vi "界面.vi"() -> ()   [LabVIEW 2024]
panel:
  in  "出错":string
  out "回答框":string
  in  "词数":dbl(slide)=50.38167938931298 scale=0.0..200.0
  in  "空白按钮":bool
  in  "发送":bool
  in  "输入框":string
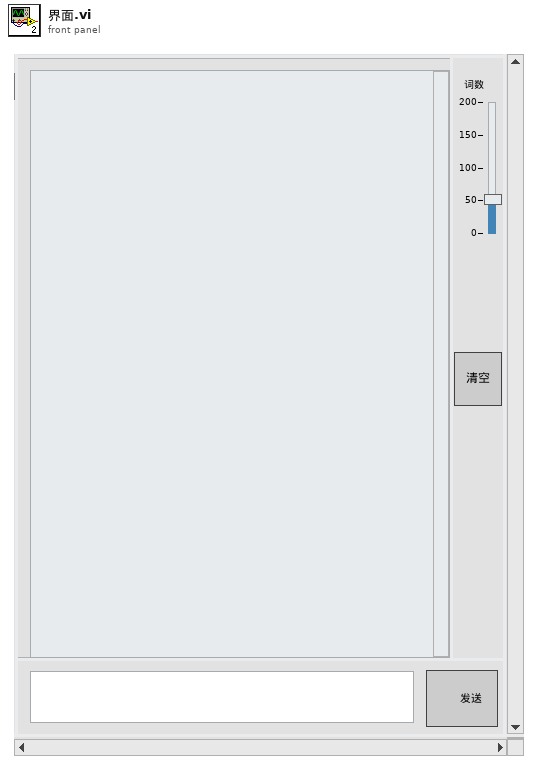
[diagram p1: front panel]
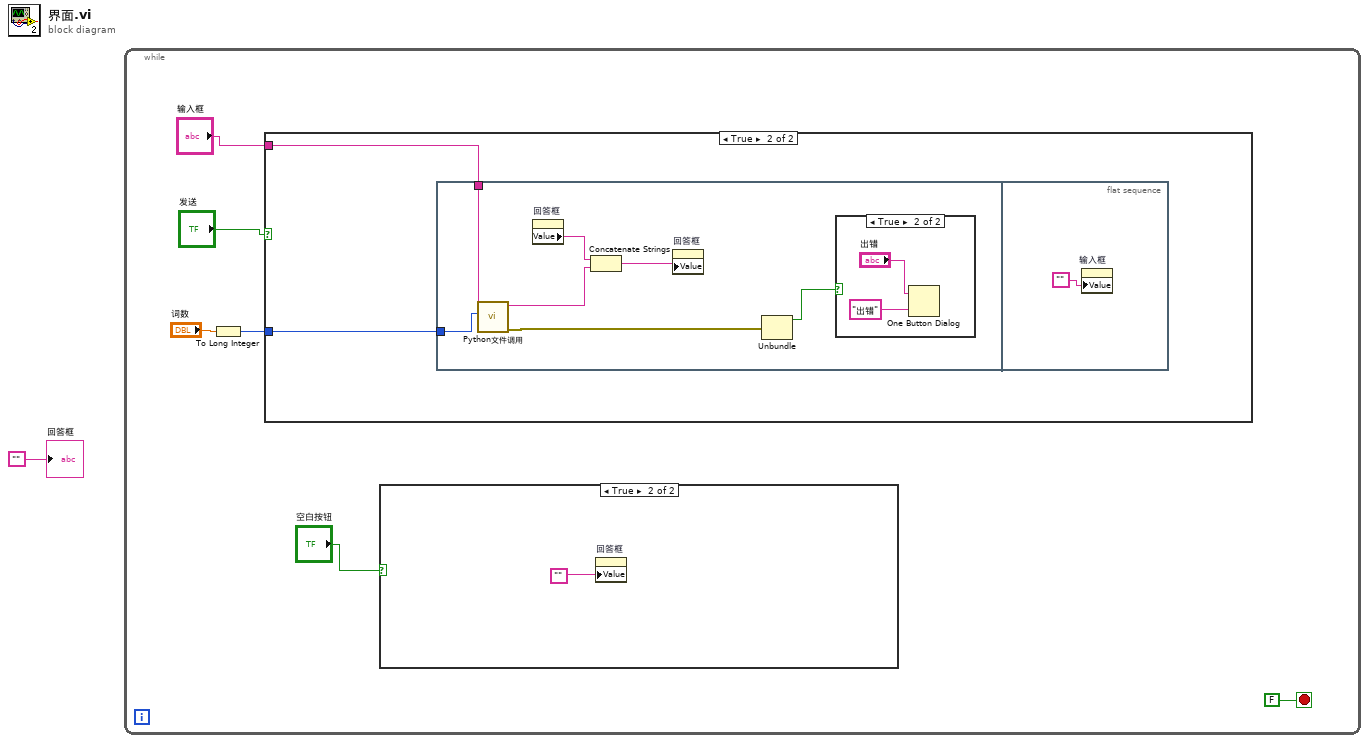
[diagram p0: block diagram]
diagram:
  n1 = while {
    stop <- FALSE stop-if-true
    n2 = To Long Integer(number="词数") -> (32bit integer=w2:i32)
    n3 = case shown="True" "发送" {
      tunnel: "输入框" -> [_ w10]
      tunnel: w2 -> [_ w9]
      frame False {
      }
      frame True {
        n4 = flat-sequence {
          tunnel: w10 -> [w17]
          tunnel: w9 -> [w11]
          frame #0 {
            n5 = call "Python文件调用.vi"("max_new_tokens"=w11, "text"=w17) -> ("错误输出"=w16:errorcluster, "out"=w13:string)  [unwired: 8 in]
            n6 = property on="回答框" class="Str"() -> ("Value"=w14:string)  [unwired: 2 in, 2 out]
            n7 = Concatenate Strings(w14, w13) -> (w12:string)
            n8 = property on="回答框" class="Str"("Value"=w12) -> ()  [unwired: 2 in, 2 out]
            n9 = Unbundle(w16) -> ("status"=w15:bool)  [unwired: 2 out]
            n10 = case shown="True" w15 {
              frame False {
              }
              frame True {
                n11 = One Button Dialog(message="出错", button name ("OK")="出错") -> ()  [unwired: 1 out]
              }
            }
          }
          frame #1 {
            n12 = property on="输入框" class="Str"("Value"="") -> ()  [unwired: 2 in, 2 out]
          }
        }
      }
    }
    n13 = case shown="True" "空白按钮" {
      frame False {
      }
      frame True {
        n14 = property on="回答框" class="Str"("Value"="") -> ()  [unwired: 2 in, 2 out]
      }
    }
  }
  "回答框" <- ""
